vi "CheckFor8bitDepth.vi"(3 "Image in":T1 {"Dialogs" format="%.0b"}) -> (0 "Success?":bool)   [LabVIEW 2024]
doc: "This VI returns a boolean value depending upon whether the image input is 8 bit or not. It also throws an error message to user."
uses:
  <userlib>/ImageProcessing/QTLIB_2595_LV86/QT_Image.ctl
  <userlib>/ImageProcessing/CameraGlobals.vi
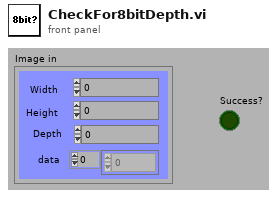
[diagram p1: front panel]
types:
  T1 = typedef "QT_Image.ctl" = cluster{"Width":i32, "Height":i32, "Depth":i32, "data":u8[], "Compressed data":u8[], "Color table":u32[], "Duration":i32, "Options":i32, "Timestamp":i32, "ID":i32, "Reserved":i32, "Dialogs":u32}
  T2 = typedef "QT_Ref.ctl" = refnum<k1>
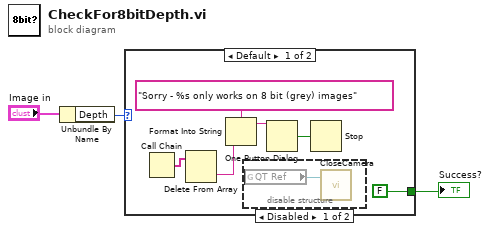
[diagram p0: block diagram]
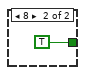
[diagram p3: hidden frame]
diagram:
  n1 = Unbundle By Name("Image in") -> ("Depth"=w2:i32)
  n2 = case shown="Default" w2 {
    tunnel: [FALSE TRUE] -> w1
    frame Default {
      n3 = Call Chain() -> (call chain=w7:string[])
      n4 = Delete From Array(array=w7) -> (deleted portion=w6:string)  [unwired: 2 in, 1 out]
      n5 = Format Into String(format string="Sorry - %s only works on 8 bit (grey) images" ("message"), w6) -> (resulting string=w8:string)  [unwired: 2 in, 1 out]
      n6 = disable-structure shown="Disabled" {
        frame Disabled {
          n7 = global read "CameraGlobals.vi" "QT Ref"() -> (w10:T2)
          n8 = call <userlib>:"CloseCamera.vi"("QT Ref In"=w10) -> ()  [unwired: 2 in, 1 out]
        }
        frame Enabled {
        }
      }
      n9 = One Button Dialog(message=w8) -> (true=w4:bool)  [unwired: 1 out]
      n10 = Stop(stop? (T)=w4) -> ()
    }
    frame 8 {
    }
  }
  "Success?" <- w1
